vi "depth sensor decode.vi"(1 "Depth Offset":dbl=10.0, 2 "Input pressure":dbl) -> (0 "Depth in m":dbl)   [LabVIEW 2021]
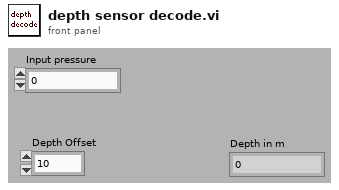
[diagram p1: front panel]
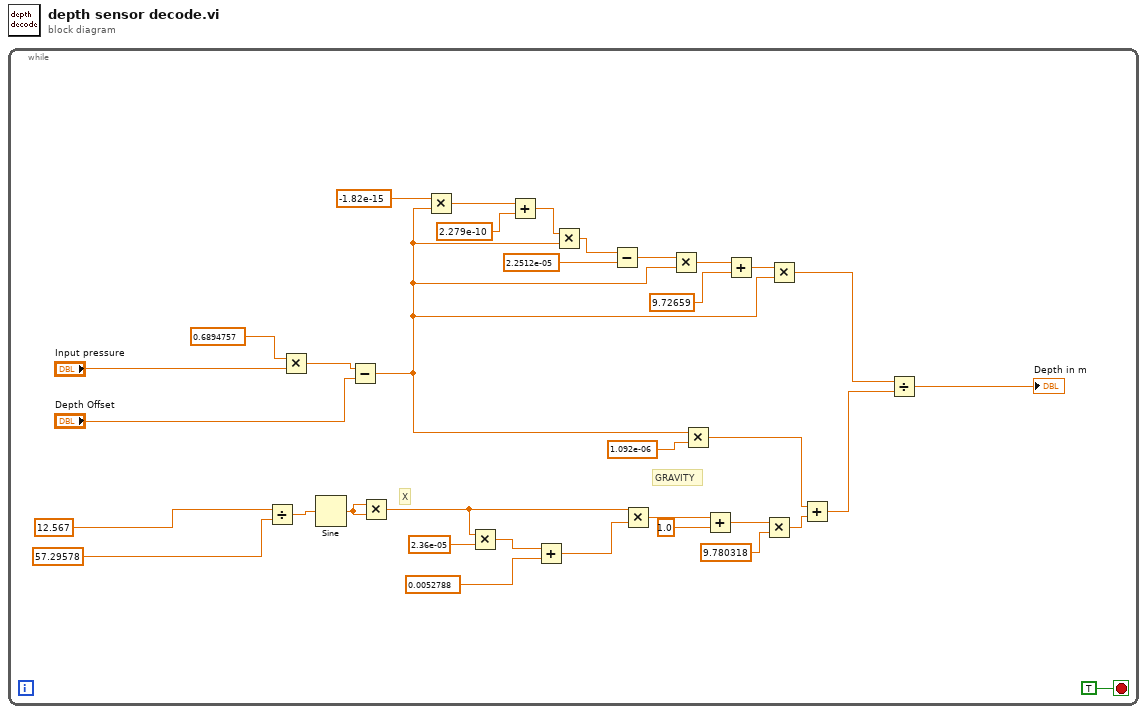
[diagram p0: block diagram]
diagram:
  n1 = while {
    stop <- TRUE stop-if-true
    # "X"
    # "GRAVITY"
    n2 = Divide(x=12.567 ("Latitute in dB"), y=57.29578) -> (x/y=w34:dbl)
    n3 = Multiply(x=0.6894757, y="Input pressure") -> (x*y=w23:dbl)
    n4 = Sine(x=w34) -> (sin(x)=w33:dbl)
    n5 = Subtract(x=w23, y="Depth Offset") -> (x-y=w9:dbl)
    n6 = Multiply(x=w33, y=w33) -> (x*y=w2:dbl)
    n7 = Multiply(x=-1.82e-15 ("y"), y=w9) -> (x*y=w17:dbl)
    n8 = Multiply(x=w2, y=2.36e-05) -> (x*y=w30:dbl)
    n9 = Add(x=w17, y=2.279e-10) -> (x+y=w16:dbl)
    n10 = Add(x=w30, y=0.0052788) -> (x+y=w29:dbl)
    n11 = Multiply(x=w16, y=w9) -> (x*y=w15:dbl)
    n12 = Subtract(x=w15, y=2.2512e-05) -> (x-y=w13:dbl)
    n13 = Multiply(x=w2, y=w29) -> (x*y=w28:dbl)
    n14 = Multiply(x=w13, y=w9) -> (x*y=w12:dbl)
    n15 = Multiply(x=w9, y=1.092e-06) -> (x*y=w20:dbl)
    n16 = Add(x=w28, y=1.0) -> (x+y=w26:dbl)
    n17 = Add(x=w12, y=9.72659) -> (x+y=w10:dbl)
    n18 = Multiply(x=w26, y=9.780318) -> (x*y=w19:dbl)
    n19 = Multiply(x=w10, y=w9) -> (x*y=w8:dbl)
    n20 = Add(x=w20, y=w19) -> (x+y=w4:dbl)
    n21 = Divide(x=w8, y=w4) -> (x/y=→"Depth in m":dbl)
  }
